vi "RSZVB Set Noise Figure LO Oscillator.vi"(8 "error in (no error)":errorcluster {"code" format="%.0x"}, 9 "LO Oscillator (Off  (0)":bool, 10 "Channel (1)":i32=1, 11 "VISA session":refnum<visa-resource-name>) -> (0 "error out":errorcluster {"code" format="%.0x"}, 3 "dup VISA session":refnum<visa-resource-name>)   [LabVIEW 2011]
doc: "This VI sets whether the analyzer assumes an ideal T0 source noise. \n\nNote(s):\n\n(1) This VI is available only with option R&S ZVAB-K30.\n\nRemote-control command(s):\n[SENSe<Ch>:]NFIGure:ISNoise ON | OFF"
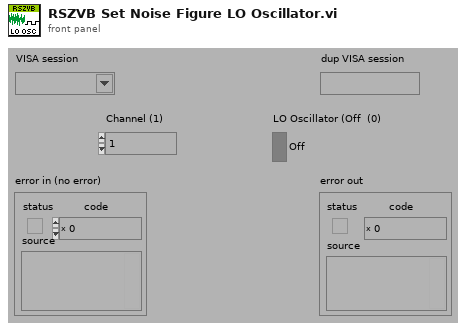
[diagram p1: front panel]
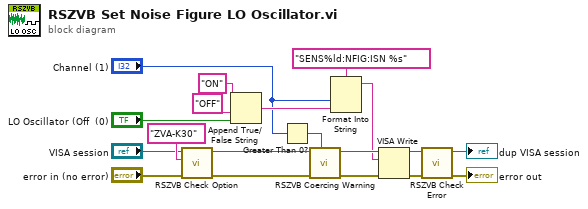
[diagram p0: block diagram]
diagram:
  n1 = call "RSZVB Check Option.vi"("error in (no error)"="error in (no error)", "Options"="ZVA-K30", "VISA session"="VISA session") -> ("error out"=w19:errorcluster, "dup VISA session"=w18:refnum<visa-resource-name>)  [unwired: 7 in]
  n2 = Append True/False String(1:"LO Oscillator (Off  (0)", 2:"OFF" ("false string"), 3:"ON" ("true string")) -> (0:w17:string)  [unwired: 1 in]
  n3 = Greater Than 0?(x="Channel (1)") -> (x > 0?=w9:bool)
  n4 = call "RSZVB Coercing Warning.vi"("In Range?"=w9, "error in (no error)"=w19, "VISA session"=w18) -> ("error out"=w10:errorcluster, "dup VISA session"=w11:refnum<visa-resource-name>)  [unwired: 7 in]
  n5 = Format Into String(format string="SENS%ld:NFIG:ISN %s", "Channel (1)", w17) -> (resulting string=w8:string)  [unwired: 2 in, 1 out]
  n6 = VISA Write(VISA resource name=w11, write buffer=w8, error in (no error)=w10) -> (VISA resource name out=w14:refnum<visa-resource-name>, error out=w13:errorcluster)  [unwired: 1 out]
  n7 = call "RSZVB Check Error.vi"("error in (no error)"=w13, "VISA session"=w14) -> ("error out"=→"error out":errorcluster, "dup VISA session"=→"dup VISA session":refnum<visa-resource-name>)  [unwired: 8 in]
